vi "add PID to engine.vi"(7 "index":i32, 8 "error in (no error)":errorcluster, 9 "PID element in":T1, 10 "engine configuration":refnum<class "engine configuration.lvclass">, 11 "Tagbus PID Module configuration in":refnum<class "PID Module configuration.lvclass">) -> (0 "error out":errorcluster, 2 "engine configuration out":refnum<class "engine configuration.lvclass">, 3 "Tagbus PID Module configuration out":refnum<class "PID Module configuration.lvclass">)   [LabVIEW 2015, in "PID Module editor node.lvclass"]
doc: "This VI adds a PID Loop to the engine"
uses:
  PID Module editor node.lvclass
  <vilib>/NI/Module Execution Interface/Engine Configuration/engine configuration.lvclass
  module/configuration/PID Module configuration.lvclass
  PID array element.ctl
  <vilib>/NI/Configuration Framework/serializable configuration/NISE_CEF_serializable configuration.lvclass/NISE_CEF_serializable configuration.ctl
  <vilib>/Utility/LVClass/Get LV Class Name.vi
  <vilib>/NI/Configuration Framework/error generator/NISE_error generator.vi
  <vilib>/NI/Configuration Framework/serializable configuration/NISE_CEF_serializable configuration.lvclass
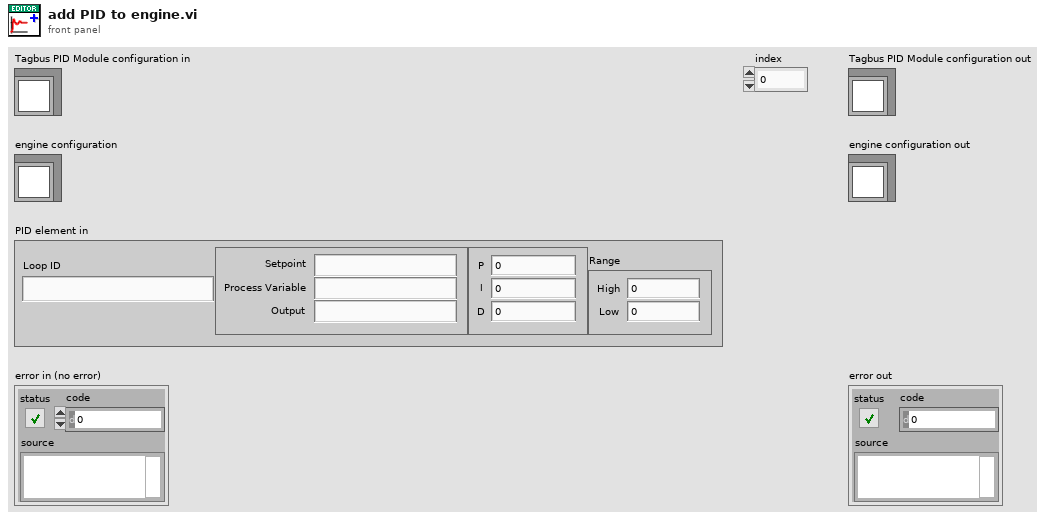
[diagram p1: front panel]
types:
  T1 = typedef "PID Module configuration.lvclass/PID array element.ctl" = cluster{"Loop ID":string, "Tags":cluster{"Setpoint":string, "Process Variable":string, "Output":string}, "Gains":cluster{"P":dbl, "I":dbl, "D":dbl}, "Range":cluster{"High":dbl, "Low":dbl}}
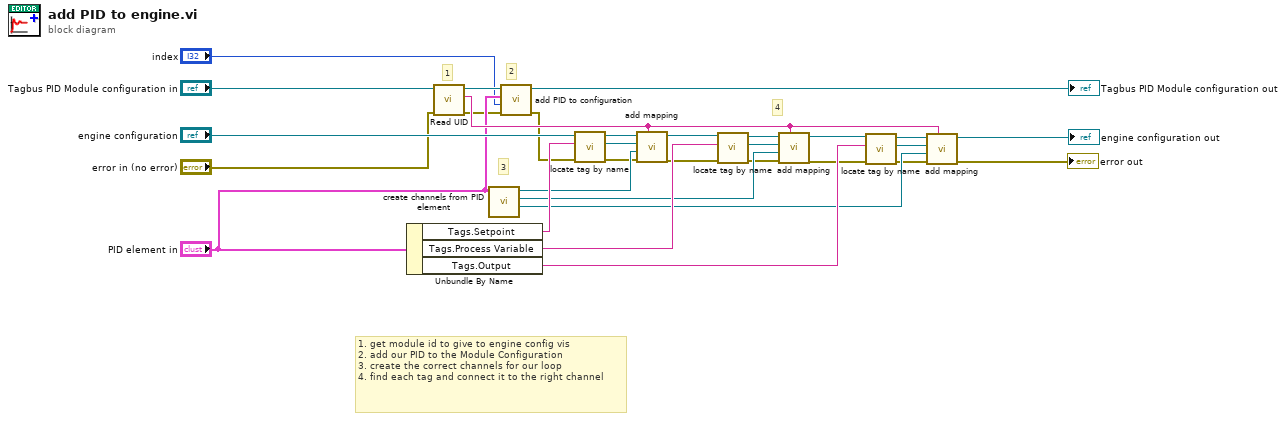
[diagram p0: block diagram]
diagram:
  # "1. get module id to give to engine config vis\n2. add our PID to the Module Configuration\n3. create the correct channels for our loop\n4. find each tag and connect it to the right channel"
  # "4"
  # "3"
  # "2"
  # "1"
  n1 = Unbundle By Name("PID element in") -> ("Tags.Setpoint"=w26:string, "Tags.Process Variable"=w28:string, "Tags.Output"=w29:string)
  n2 = call <vilib>:"Read UID.vi"("error in"="error in (no error)", "configuration in"="Tagbus PID Module configuration in") -> ("error out"=w12:errorcluster, "instance id"=w21:string, "configuration out"=w18:refnum<class "PID Module configuration.lvclass">)  [unwired: 7 in]
  n3 = call "create channels from PID element.vi"("line item in"="PID element in") -> ("Output Channel Out"=w22:refnum<class "TBM channel.lvclass">, "Process Variable Channel Out"=w24:refnum<class "TBM channel.lvclass">, "Setpoint Channel Out"=w23:refnum<class "TBM channel.lvclass">)  [unwired: 8 in]
  n4 = call "add PID to configuration.vi"("error in"=w12, "index"="index", "PID Element in"="PID element in", "Tagbus PID Module configuration in"=w18) -> ("error out"=w11:errorcluster, "Tagbus PID Module configuration out"=→"Tagbus PID Module configuration out":refnum<class "PID Module configuration.lvclass">)  [unwired: 6 in]
  n5 = call <vilib>:"locate tag by name.vi"("error in"=w11, "tag name"=w26, "engine configuration in"="engine configuration") -> ("error out"=w13:errorcluster, "tag descriptor"=w27:refnum<class "tag descriptor.lvclass">, "engine configuration out"=w9:refnum<class "engine configuration.lvclass">)  [unwired: 6 in]
  n6 = call <vilib>:"add mapping.vi"("owner ID"=w21, "error in"=w13, "channel"=w23, "tag descriptor"=w27, "engine configuration"=w9) -> ("error out"=w3:errorcluster, "engine configuration out"=w8:refnum<class "engine configuration.lvclass">)  [unwired: 5 in]
  n7 = call <vilib>:"locate tag by name.vi"("error in"=w3, "tag name"=w28, "engine configuration in"=w8) -> ("error out"=w15:errorcluster, "tag descriptor"=w30:refnum<class "tag descriptor.lvclass">, "engine configuration out"=w7:refnum<class "engine configuration.lvclass">)  [unwired: 6 in]
  n8 = call <vilib>:"add mapping.vi"("owner ID"=w21, "error in"=w15, "channel"=w24, "tag descriptor"=w30, "engine configuration"=w7) -> ("error out"=w4:errorcluster, "engine configuration out"=w6:refnum<class "engine configuration.lvclass">)  [unwired: 5 in]
  n9 = call <vilib>:"locate tag by name.vi"("error in"=w4, "tag name"=w29, "engine configuration in"=w6) -> ("error out"=w14:errorcluster, "tag descriptor"=w31:refnum<class "tag descriptor.lvclass">, "engine configuration out"=w5:refnum<class "engine configuration.lvclass">)  [unwired: 6 in]
  n10 = call <vilib>:"add mapping.vi"("owner ID"=w21, "error in"=w14, "channel"=w22, "tag descriptor"=w31, "engine configuration"=w5) -> ("error out"=→"error out":errorcluster, "engine configuration out"=→"engine configuration out":refnum<class "engine configuration.lvclass">)  [unwired: 5 in]
